vi "Lecture Param.vi"(8 "errin":errorcluster) -> (0 "error out":errorcluster caption="errout")   [LabVIEW 2020]
uses:
  <vilib>/Utility/config.llb/Read Key (Double).vi
  <vilib>/Utility/config.llb/Read Key (String).vi
  Param.vi
  <vilib>/Utility/config.llb/NI_LVConfig.lvlib
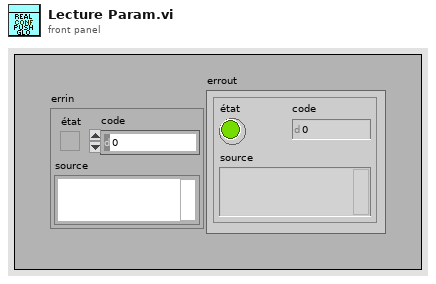
[diagram p1: front panel]
types:
  T1 = typedef "NI_LVConfig.lvlib/Config Data RefNum.ctl" = refnum<k1>
  T2 = cluster{"[0]":string, "[1]":string, "[2]":string, "[3]":string, "[4]":string}
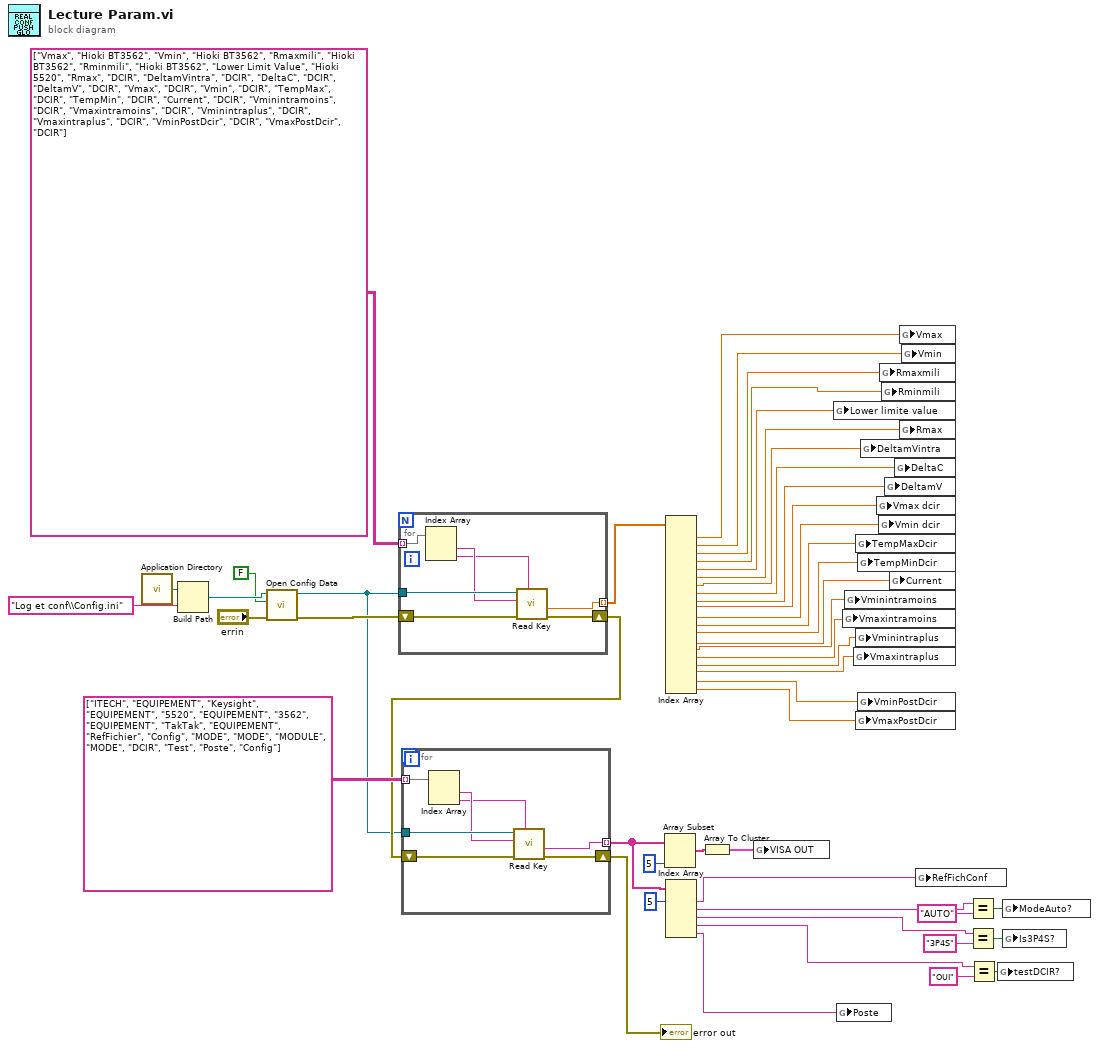
[diagram p0: block diagram]
diagram:
  n1 = call <vilib>:"Application Directory.vi"() -> ("Application Directory"=w23:path)
  n2 = Build Path(base path=w23, name or relative path="Log et conf\\Config.ini") -> (appended path=w47:path)
  n3 = call <vilib>:"Open Config Data.vi"("error in (no error)"="errin", "create file if necessary (T)"=FALSE, "configuration file path"=w47) -> ("error out"=w45:errorcluster, "refnum"=w19:T1)  [unwired: 6 in, 1 out]
  n4 = for {
    tunnel: w19 -> [w54]
    tunnel: string[][] [["Vmax", "Hioki BT3562"], ["Vmin", "Hioki BT3562"], ["Rmaxmili", "Hioki BT3562"], ["Rminmili", "Hioki BT3562"], ["Lower Limit Value", "Hioki 5520"], ["Rmax", "DCIR"], ["DeltamVintra", "DCIR"], ["DeltaC", "DCIR"], ["DeltamV", "DCIR"], ["Vmax", "DCIR"], ["Vmin", "DCIR"], ["TempMax", "DCIR"], ["TempMin", "DCIR"], ["Current", "DCIR"], ["Vminintramoins", "DCIR"], ["Vmaxintramoins", "DCIR"], ["Vminintraplus", "DCIR"], ["Vmaxintraplus", "DCIR"], ["VminPostDcir", "DCIR"], ["VmaxPostDcir", "DCIR"]] -> [w53] mode=indexing
    shift-right: [w50] -> w21
    shift-left: w45 -> [w55]
    tunnel: [w49] -> w42 mode=indexing
    n5 = Index Array(array=w53) -> (element #1=w52:string, element #2=w51:string)  [unwired: 2 in]
    n6 = call-poly <vilib>:"Read Key.vi"("section"=w51, "error in (no error)"=w55, "key"=w52, "refnum"=w54) -> ("error out"=w50:errorcluster, "value"=w49:dbl)  [unwired: 4 in, 2 out]
  }
  n7 = for {
    tunnel: w19 -> [w61]
    tunnel: string[][] [["ITECH", "EQUIPEMENT"], ["Keysight", "EQUIPEMENT"], ["5520", "EQUIPEMENT"], ["3562", "EQUIPEMENT"], ["TakTak", "EQUIPEMENT"], ["RefFichier", "Config"], ["MODE", "MODE"], ["MODULE", "MODE"], ["DCIR", "Test"], ["Poste", "Config"]] -> [w60] mode=indexing
    shift-right: [w57] -> w20
    shift-left: w21 -> [w62]
    tunnel: [w56] -> w13 mode=indexing
    n8 = Index Array(array=w60) -> (element #1=w59:string, element #2=w58:string)  [unwired: 2 in]
    n9 = call-poly <vilib>:"Read Key.vi"("section"=w58, "error in (no error)"=w62, "key"=w59, "refnum"=w61) -> ("error out"=w57:errorcluster, "value"=w56:string)  [unwired: 4 in, 2 out]
  }
  "error out" <- w20
  n10 = Array Subset(array=w13, length=5 ("longueur")) -> (w17:string[])  [unwired: 1 in]
  n11 = Index Array(array=w42) -> (element #1=w41:dbl, element #2=w40:dbl, element #3=w39:dbl, element #4=w38:dbl, element #5=w37:dbl, element #6=w36:dbl, element #7=w35:dbl, element #8=w34:dbl, element #9=w33:dbl, element #10=w32:dbl, element #11=w31:dbl, element #12=w30:dbl, element #13=w29:dbl, element #14=w28:dbl, element #15=w27:dbl, element #16=w26:dbl, element #17=w25:dbl, element #18=w24:dbl, element #19=w3:dbl, element #20=w2:dbl)  [unwired: 20 in]
  n12 = Index Array(array=w13, index #1=5 ("indice")) -> (element #1=w14:string, element #2=w12:string, element #3=w11:string, element #4=w4:string, element #5=w1:string)  [unwired: 4 in]
  n13 = Array To Cluster(array=w17) -> (cluster=w18:T2)
  n14 = global write "Param.vi" "VISA OUT"(w18) -> ()
  n15 = global write "Param.vi" "Lower limite value"(w37) -> ()
  n16 = global write "Param.vi" "Poste"(w1) -> ()
  n17 = global write "Param.vi" "Vmaxintramoins"(w26) -> ()
  n18 = global write "Param.vi" "Vminintramoins"(w27) -> ()
  n19 = global write "Param.vi" "Vmaxintraplus"(w24) -> ()
  n20 = global write "Param.vi" "TempMaxDcir"(w30) -> ()
  n21 = global write "Param.vi" "Vminintraplus"(w25) -> ()
  n22 = global write "Param.vi" "VmaxPostDcir"(w2) -> ()
  n23 = global write "Param.vi" "TempMinDcir"(w29) -> ()
  n24 = global write "Param.vi" "VminPostDcir"(w3) -> ()
  n25 = global write "Param.vi" "DeltamVintra"(w35) -> ()
  n26 = global write "Param.vi" "Vmax dcir"(w32) -> ()
  n27 = global write "Param.vi" "Vmin dcir"(w31) -> ()
  n28 = global write "Param.vi" "Rmaxmili"(w39) -> ()
  n29 = global write "Param.vi" "Rminmili"(w38) -> ()
  n30 = global write "Param.vi" "DeltamV"(w33) -> ()
  n31 = global write "Param.vi" "Current"(w28) -> ()
  n32 = global write "Param.vi" "DeltaC"(w34) -> ()
  n33 = global write "Param.vi" "Vmax"(w41) -> ()
  n34 = global write "Param.vi" "Rmax"(w36) -> ()
  n35 = global write "Param.vi" "Vmin"(w40) -> ()
  n36 = global write "Param.vi" "RefFichConf"(w14) -> ()
  n37 = Equal? ("Égaux ?")(x=w12, y="AUTO") -> (x = y?=w10:bool)
  n38 = Equal? ("Égaux ?")(x=w11, y="3P4S") -> (x = y?=w9:bool)
  n39 = Equal? ("Égaux ?")(x=w4, y="OUI") -> (x = y?=w6:bool)
  n40 = global write "Param.vi" "testDCIR?"(w6) -> ()
  n41 = global write "Param.vi" "ModeAuto?"(w10) -> ()
  n42 = global write "Param.vi" "Is3P4S?"(w9) -> ()
